vi "Get flattened data.vi"(8 "error in (no error)":errorcluster, 11 "Bool D Element in":refnum<class "Bool D Element.lvclass">) -> (0 "error out":errorcluster, 2 "Flattened data":u8[](array[numeric]), 3 "Bool D Element out":refnum<class "Bool D Element.lvclass">)   [LabVIEW 2018, in "D Datagrid Library.lvlib" / "Bool D Element.lvclass"]
uses:
  Bool D Element.lvclass
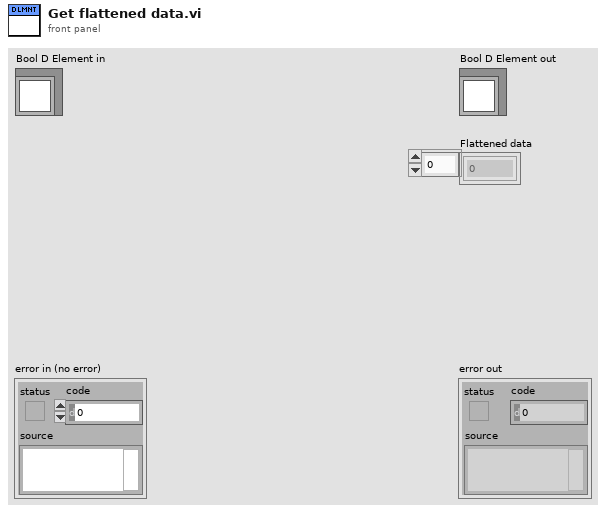
[diagram p1: front panel]
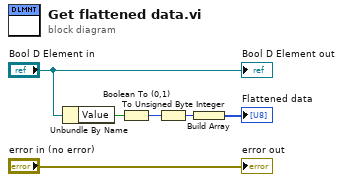
[diagram p0: block diagram]
diagram:
  n1 = Unbundle By Name("Bool D Element in") -> ("Value"=w4:bool)
  n2 = Boolean To (0,1)(Boolean=w4) -> (0, 1=w3:i16)
  n3 = To Unsigned Byte Integer(number=w3) -> (unsigned 8bit integer=w2:u8)
  n4 = Build Array(w2) -> (→"Flattened data":u8[])
  "error out" <- "error in (no error)"
  "Bool D Element out" <- "Bool D Element in"
